vi "case_move.vi"(7 "Uninitialized message":string, 8 "error in (no error)":errorcluster, 9 "initialized":bool, 10 "message cluster":T1, 11 "VISA Refnum in":refnum<visa-resource-name>) -> (0 "error out":errorcluster, 3 "VISA Refnum out":refnum<visa-resource-name>)   [LabVIEW 2020]
uses:
  controls/message cluster.ctl
  <instrlib>/Marlin Instrument Driver/Public/controls/move parameters.ctl
  <instrlib>/Marlin Instrument Driver/Marlin Instrument Driver.lvlib
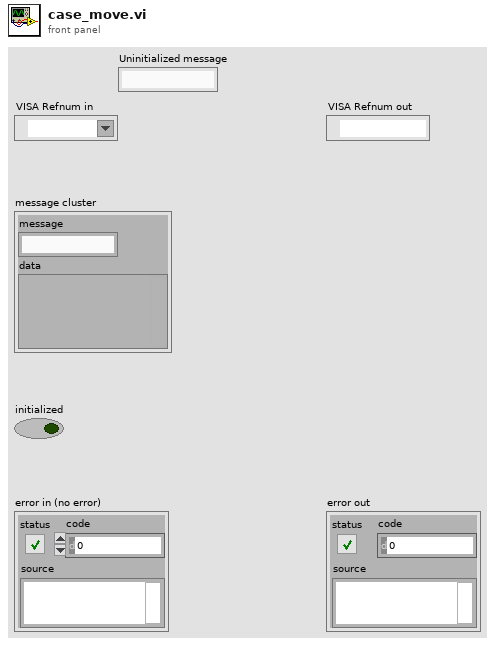
[diagram p1: front panel]
types:
  T1 = typedef "message cluster.ctl" = cluster{"message":string, "data":variant}
  T2 = typedef "Marlin Instrument Driver.lvlib/move parameters.ctl" = cluster{"E":dbl, "F":dbl, "X":dbl, "Y":dbl, "Z":dbl}
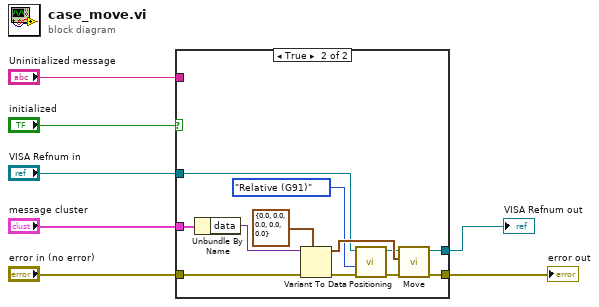
[diagram p0: block diagram]
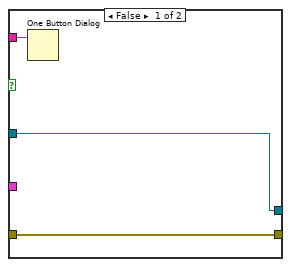
[diagram p2: hidden frame]
diagram:
  n1 = case shown="True" "initialized" {
    tunnel: "message cluster" -> [_ w22]
    tunnel: [w10 w18] -> w2
    tunnel: "error in (no error)" -> [w10 w17]
    tunnel: [w9 w16] -> w4
    tunnel: "VISA Refnum in" -> [w9 w13]
    tunnel: "Uninitialized message" -> [w8 _]
    frame False {
      n2 = One Button Dialog(message=w8) -> ()  [unwired: 1 in, 1 out]
    }
    frame True {
      n3 = Unbundle By Name(w22) -> ("data"=w21:variant)
      n4 = Variant To Data(error in=w17, type=T2 {"E"=0.0, "F"=0.0, "X"=0.0, "Y"=0.0, "Z"=0.0} ("Distances"), Variant=w21) -> (data=w19:T2, error out=w15:errorcluster)
      n5 = call <instrlib>:"Positioning.vi"("error in (no error)"=w15, "type"=enum16{"Absolute (G90)", "Relative (G91)"}."Relative (G91)", "VISA resource name"=w13) -> ("error out"=w14:errorcluster, "VISA resource name out"=w12:refnum<visa-resource-name>)  [unwired: 7 in]
      n6 = call <instrlib>:"Move.vi"("error in (no error)"=w14, "Distances"=w19, "VISA resource name"=w12) -> ("error out"=w18:errorcluster, "VISA resource name out"=w16:refnum<visa-resource-name>)  [unwired: 7 in]
    }
  }
  "VISA Refnum out" <- w4
  "error out" <- w2
